vi "SpinIntake.vi"(8 "Error In":errorcluster, 9 "Time":dbl, 10 "Initation?":bool, 11 "Speed":dbl) -> (0 "Error Out":errorcluster, 3 "Finished":bool)   [LabVIEW 2020]
uses:
  <vilib>/Utility/semaphor.llb/Obtain Semaphore Reference.vi
  <vilib>/Rock Robotics/WPI/ThirdParty/JAS_Junk/TrajLib/Timer_Reset.vi
  AuxGlobals.vi
  <vilib>/Rock Robotics/WPI/ThirdParty/JAS_Junk/TrajLib/Trajectory_Library.lvlib
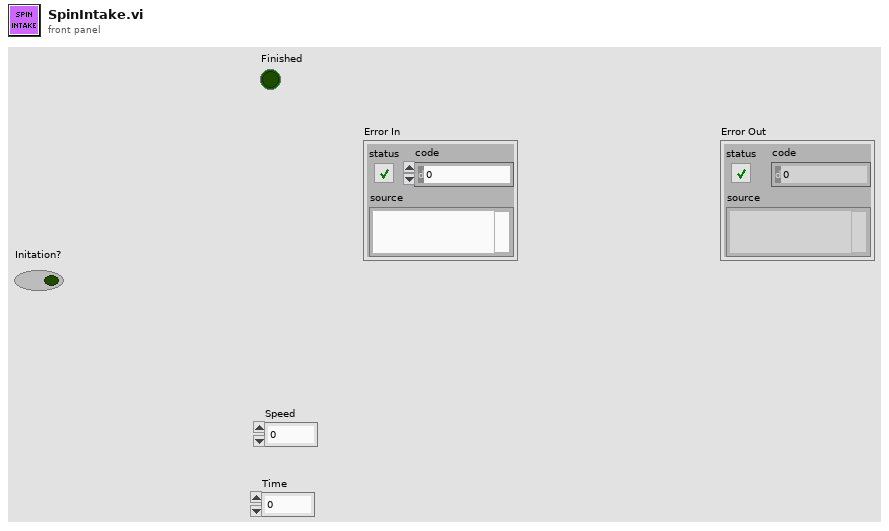
[diagram p1: front panel]
types:
  T1 = typedef "Trajectory_Library.lvlib/TIMER.ctl" = cluster{"StartTime":dbl, "Accumulated TIme":dbl, "Running":bool, "semaphore":T2}
  T2 = typedef "Semaphore RefNum" = refnum<k1>
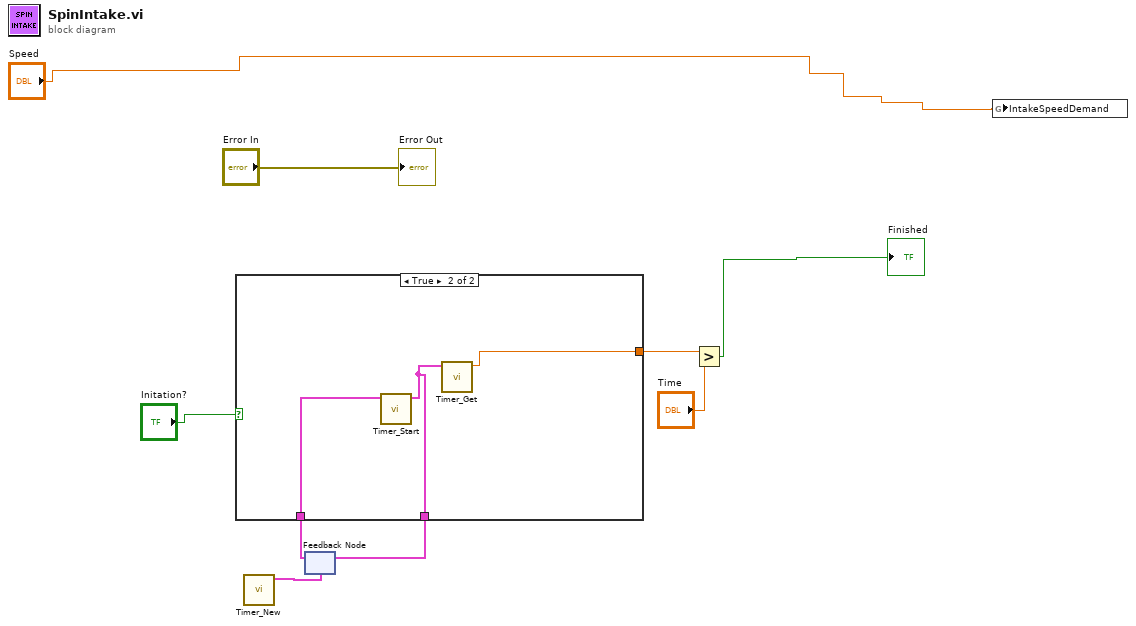
[diagram p0: block diagram]
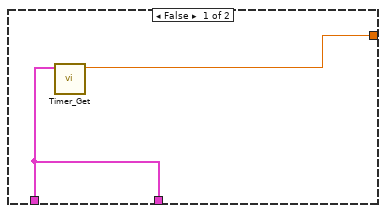
[diagram p2: hidden frame]
diagram:
  n1 = call <vilib>:"Timer_New.vi"() -> ("TIMER"=w5:T1)  [unwired: 11 in]
  n2 = feedback #1(w5) -> (w7:T1)
  n3 = case shown="True" "Initation?" {
    tunnel: w7 -> [w10 w13]
    tunnel: [w11 w14] -> w6
    tunnel: [w10 w12] -> w4
    frame False {
      n4 = call <vilib>:"Timer_Get.vi"("TIMER"=w10) -> ("CurrentTImer"=w11:dbl)  [unwired: 10 in]
    }
    frame True {
      n5 = call <vilib>:"Timer_Start.vi"("in Timer"=w13) -> ("out Timer"=w12:T1)  [unwired: 10 in]
      n6 = call <vilib>:"Timer_Get.vi"("TIMER"=w12) -> ("CurrentTImer"=w14:dbl)  [unwired: 10 in]
    }
  }
  n7 = feedback-in #1(w4) -> ()
  n8 = Greater?(x=w6, y="Time") -> (0:→"Finished":bool)
  n9 = global write "AuxGlobals.vi" "IntakeSpeedDemand"("Speed") -> ()
  "Error Out" <- "Error In"
